vi "RT Writer.vi"() -> ()   [LabVIEW 2018]
uses:
  <vilib>/userdefined/High Color/IMAQdx.ctl
  <vilib>/vision/driver/NI_Vision_Acquisition_Software.lvlib
panel:
  in  "stop":bool
  out "error out":errorcluster
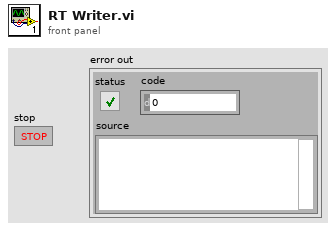
[diagram p1: front panel]
types:
  T1 = typedef "IMAQdx.ctl" = refnum<k21>
  T2 = typedef "IMAQ Image.ctl" = refnum<image>
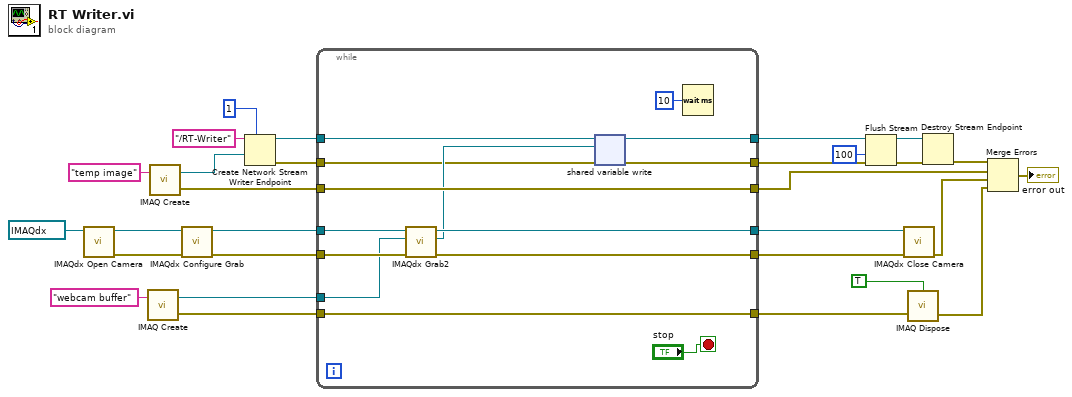
[diagram p0: block diagram]
diagram:
  n1 = call <vilib>:"IMAQdx Open Camera.vi"("Session In"=T1 "cam1") -> ("error out"=w20:errorcluster, "Session Out"=w21:T1)  [unwired: 9 in]
  n2 = call "IMAQ Create"("Image Name"="webcam buffer") -> ("New Image"=w15:T2, "error out"=w16:errorcluster)  [unwired: 4 in]
  n3 = call "IMAQ Create"("Image Name"="temp image") -> ("New Image"=w26:T2, "error out"=w23:errorcluster)  [unwired: 4 in]
  n4 = call <vilib>:"IMAQdx Configure Grab.vi"("error in"=w20, "Session In"=w21) -> ("error out"=w17:errorcluster, "Session Out"=w19:T1)  [unwired: 8 in]
  n5 = Create Network Stream Writer Endpoint(7:1 ("writer buffer size"), 9:w26, 11:"/RT-Writer" ("writer name")) -> (0:w24:errorcluster, 3:w25:refnum<k21>)  [unwired: 4 in]
  n6 = while {
    tunnel: w25 -> [w36]
    tunnel: w24 -> [w34]
    tunnel: w23 -> [w39]
    tunnel: w19 -> [w43]
    tunnel: [w42] -> w18
    tunnel: w17 -> [w41]
    tunnel: [w40] -> w8
    tunnel: [w39] -> w6
    tunnel: w16 -> [w38]
    tunnel: [w38] -> w10
    tunnel: w15 -> [w37]
    tunnel: [w33] -> w14
    tunnel: [w32] -> w12
    stop <- "stop" stop-if-true
    n7 = call <vilib>:"IMAQdx Grab2.vi"("error in"=w41, "Image In"=w37, "Session In"=w43) -> ("error out"=w40:errorcluster, "Image Out"=w35:T2, "Session Out"=w42:T1)  [unwired: 5 in, 1 out]
    n8 = shared-variable-write(w36, w34, w35) -> (w32:refnum<k21>, w33:errorcluster)  [unwired: 1 in, 1 out]
    n9 = Wait (ms)(milliseconds to wait=u32 10) -> ()  [unwired: 1 out]
  }
  n10 = Flush Stream(8:w14, 9:100 ("timeout in ms (-1)"), 11:w12) -> (0:w13:errorcluster, 3:w11:refnum<k21>)  [unwired: 1 in, 1 out]
  n11 = call <vilib>:"IMAQdx Close Camera.vi"("error in"=w8, "Session In"=w18) -> ("error out"=w5:errorcluster)  [unwired: 9 in]
  n12 = call "IMAQ Dispose"("All Images? (No)"=TRUE, "error in (no error)"=w10) -> ("error out"=w4:errorcluster)  [unwired: 4 in]
  n13 = Destroy Stream Endpoint(8:w13, 11:w11) -> (0:w7:errorcluster)
  n14 = Merge Errors(w7, w6, w5, w4) -> (→"error out":errorcluster)
